vi "destroySound.vi"(8 "error in (no error)":errorcluster, 11 "Sound in":refnum<class "Sound.lvclass">) -> (0 "error out":errorcluster, 3 "Sound out":refnum<class "Sound.lvclass">)   [LabVIEW 2019, in "Sound.lvclass"]
uses:
  Sound.lvclass
  Sound.lvclass/Sound.ctl
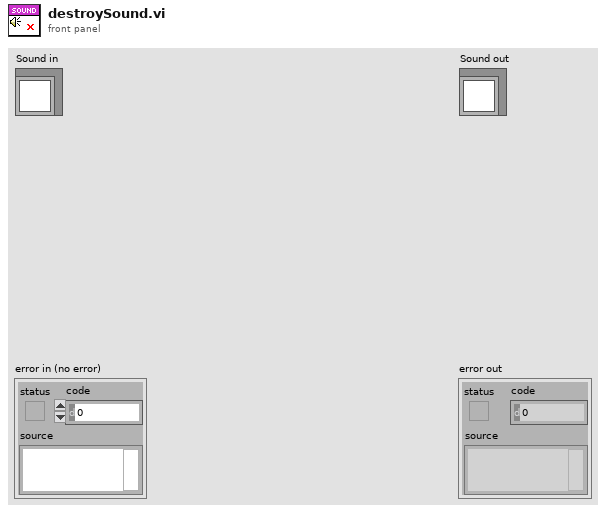
[diagram p1: front panel]
types:
  T1 = typedef "Sound Output Task ID.ctl" = u32
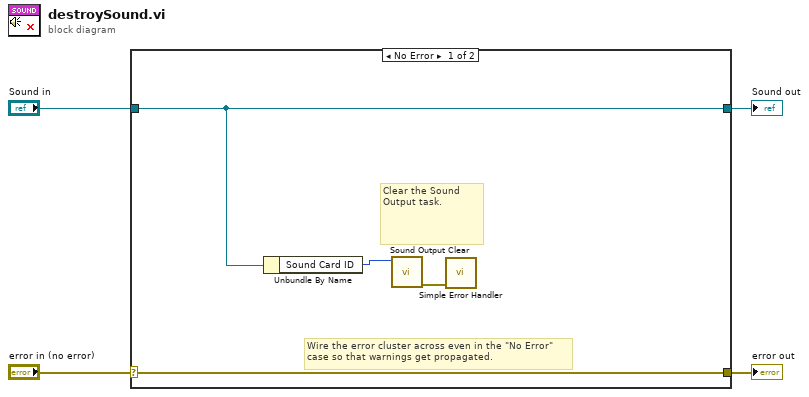
[diagram p0: block diagram]
diagram:
  n1 = case shown="No Error" "error in (no error)" {
    selector: "error in (no error)" -> [w8 w10]
    tunnel: [w8 w10] -> w3
    tunnel: [w6 w9] -> w1
    tunnel: "Sound in" -> [w6 w9]
    frame No Error {
      # "Clear the Sound Output task."
      # "Wire the error cluster across even in the \"No Error\"\ncase so that warnings get propagated."
      n2 = Unbundle By Name(w6) -> ("Sound Card ID"=w5:T1)
      n3 = call <vilib>:"Sound Output Clear.vi"("task ID"=w5) -> ("error out"=w7:errorcluster)  [unwired: 10 in]
      n4 = call <vilib>:"Simple Error Handler.vi"("error in (no error)"=w7) -> ()  [unwired: 4 in, 5 out]
    }
    frame Error {
    }
  }
  "error out" <- w3
  "Sound out" <- w1
